vi "find_patches.vi"(5 "Shrink Factor":i32=1, 6 "Field of View":cluster{"fieldOfViewX":sgl, "fieldOfViewY":sgl}, 7 "Log File Directory":string, 8 "error in":errorcluster, 9 "debug":bool, 10 "find_patches parameters":T2, 11 "Image":T3) -> (0 "error out":errorcluster, 2 "Patches":T1(array[cluster]))   [LabVIEW 2017, in "gVision.lvlib"]
uses:
  gVision.lvlib
  <vilib>/vision/Image Controls.llb/IMAQ Image.ctl
  find_patches parameters.ctl
panel:
  # "Image must be an 8-bin greyscale image"
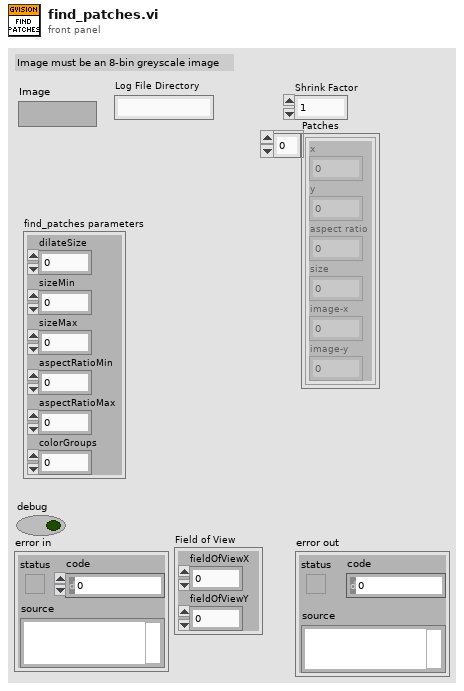
[diagram p1: front panel]
types:
  T1 = cluster{"x":dbl, "y":dbl, "aspect ratio":dbl, "size":dbl, "image-x":dbl, "image-y":dbl}[]
  T2 = typedef "find_patches parameters.ctl" = cluster{"dilateSize":i32, "sizeMin":sgl, "sizeMax":sgl, "aspectRatioMin":sgl, "aspectRatioMax":sgl, "colorGroups":i32}
  T3 = typedef "IMAQ Image.ctl" = refnum<image>
  T4 = enum32{"Map Pixel Pointer", "Unmap Pixel Pointer", "Get Pixels Infos"}
  T5 = cluster{"x":dbl, "y":dbl, "aspect ratio":dbl, "size":dbl, "image-x":dbl, "image-y":dbl}
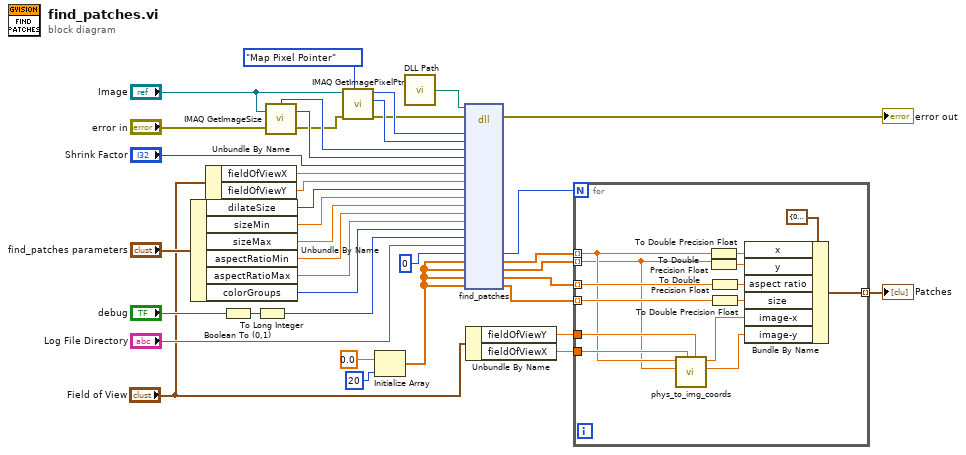
[diagram p0: block diagram]
diagram:
  n1 = Unbundle By Name("find_patches parameters") -> ("dilateSize"=w26:i32, "sizeMin"=w25:sgl, "sizeMax"=w24:sgl, "aspectRatioMin"=w23:sgl, "aspectRatioMax"=w22:sgl, "colorGroups"=w21:i32)
  n2 = Unbundle By Name("Field of View") -> ("fieldOfViewX"=w2:sgl, "fieldOfViewY"=w1:sgl)
  n3 = Boolean To (0,1)(Boolean="debug") -> (0, 1=w29:i16)
  n4 = To Long Integer(number=w29) -> (32bit integer=w28:i32)
  n5 = call "IMAQ GetImageSize"("Image"="Image", "error in (no error)"="error in") -> ("Y Resolution"=w9:i32, "X Resolution"=w10:i32, "error out"=w8:errorcluster)  [unwired: 2 in]
  n6 = call "IMAQ GetImagePixelPtr"("Function"=T4."Map Pixel Pointer", "error in (no error)"=w8, "Image"="Image") -> ("error out"=w14:errorcluster, "LineWidth(Pixels)"=w31:i32, "Pixel Pointer out"=w32:u64)  [unwired: 3 in, 3 out]
  n7 = Initialize Array(sgl 0.0 ("element"), 20 ("dimension size")) -> (w19:sgl[])
  n8 = call "DLL Path.vi"() -> ("DLL Path"=w34:path)  [unwired: 5 in]
  n9 = dll-call lib="?" fn="find_patches"(path in=w34, error in=w14, "imgPtr"=w32, "imgLineWidth"=w31, "imgWidth"=w10, "imgHeight"=w9, "shrinkFactor"="Shrink Factor", "fieldOfViewX"=w2, "fieldOfViewY"=w1, "dilateSize"=w26, "sizeMin"=w25, "sizeMax"=w24, "aspectRatioMin"=w23, "aspectRatioMax"=w22, "colorGroups"=w21, "debug"=w28, "logFileDir"="Log File Directory", "numPatches"=0 ("numFiducials"), "patchXCoordinates"=w19, "patchYCoordinates"=w19, "patchAspectRatios"=w19, "patchSizes"=w19) -> (error out=→"error out":errorcluster, "numPatches"=w27:i32, "patchXCoordinates"=w18:sgl[], "patchYCoordinates"=w17:sgl[], "patchAspectRatios"=w16:sgl[], "patchSizes"=w15:sgl[])  [unwired: 17 in, 1 out]
  n10 = Unbundle By Name("Field of View") -> ("fieldOfViewY"=w6:sgl, "fieldOfViewX"=w5:sgl)
  n11 = for {
    N: w27 -> [_]
    tunnel: w18 -> [w42] mode=indexing
    tunnel: w17 -> [w41] mode=indexing
    tunnel: [w52] -> w4 mode=indexing
    tunnel: w16 -> [w47] mode=indexing
    tunnel: w15 -> [w46] mode=indexing
    tunnel: w6 -> [w44]
    tunnel: w5 -> [w43]
    n12 = call "phys_to_img_coords.vi"("fov_y"=w44, "fov_x"=w43, "y"=w41, "x"=w42) -> ("image_y"=w39:dbl, "image_x"=w40:dbl)  [unwired: 6 in]
    n13 = To Double Precision Float(number=w42) -> (double precision float=w51:dbl)
    n14 = To Double Precision Float(number=w41) -> (double precision float=w50:dbl)
    n15 = To Double Precision Float(number=w47) -> (double precision float=w49:dbl)
    n16 = To Double Precision Float(number=w46) -> (double precision float=w48:dbl)
    n17 = Bundle By Name(cluster=T5 {"x"=0.0, "y"=0.0, "aspect ratio"=0.0, "size"=0.0, "image-x"=0.0, "image-y"=0.0}, "x"=w51, "y"=w50, "aspect ratio"=w49, "size"=w48, "image-x"=w40, "image-y"=w39) -> (w52:T5)
  }
  "Patches" <- w4
